vi "Read_Break_List.vi"(8 "error in (no error)":errorcluster, 11 "Ref in":T4={"MS SQL Connection"=refnum, "UDL File"=path "", "Time"="", "DCODE"="", "WIP+1"=0, "MC No?"=0, "POKAYOKE?"=FALSE, "Expected Result"="", "Result [Status]"="", "Clock"=0.0, "RFID"="", "WIP Queue"=refnum, "TS Parameter"={"ProfitCenterCode"="", "LineCode"="", "WorkOrderNumber"="", "Model"="", "Model_with_Prefix"="", "VendorCode"="", "SetParameterDateCode"="", "PokaYoke"=0, "Target"=1, "Live_DateCode"="", "CustomerPartNumber"="", "Hand"="", "sBarcode"=FALSE, "FCA"=0, "Ent_Stamp"=timestamp(0 s since 1904-01-01), "STS_CD"=0.0}, "Data_Queue"=[], "RFID Serial No."=""} {"TS Parameter"."FCA" format="%01d"; "TS Parameter"."Target" min=1 max=100000; "TS Parameter"."PokaYoke" min=0 max=1}) -> (0 "error out":errorcluster, 3 "Break List":T3[](array[typedef]) {"End Time" format="%<%d/%m/%Y\n%I:%M:%S %p>T"; "Start Time" format="%<%d/%m/%Y\n%I:%M:%S %p>T"}, 4 "Operator List":string[](array[string]), 6 "Breakdown List":string[](array[string]))   [LabVIEW 2020]
uses:
  Controls/TD SQL.ctl
  <vilib>/addons/database/Connection.llb/Conn ObjectReference.ctl
  Controls/WIP_State.ctl
  Controls/TS_Parameter.ctl
  Controls/Breakdown_List.ctl
  Controls/Loss_type.ctl
  <vilib>/addons/database/_DB Variant To Data/Database Variant To Data.xnode
  <vilib>/addons/database/NI_Database_API.lvlib
panel:
  out "data 2":string[][](array[string])
  out "f":T1
  out "data":string[](array[string])
  in  "Machine":T2(ring)
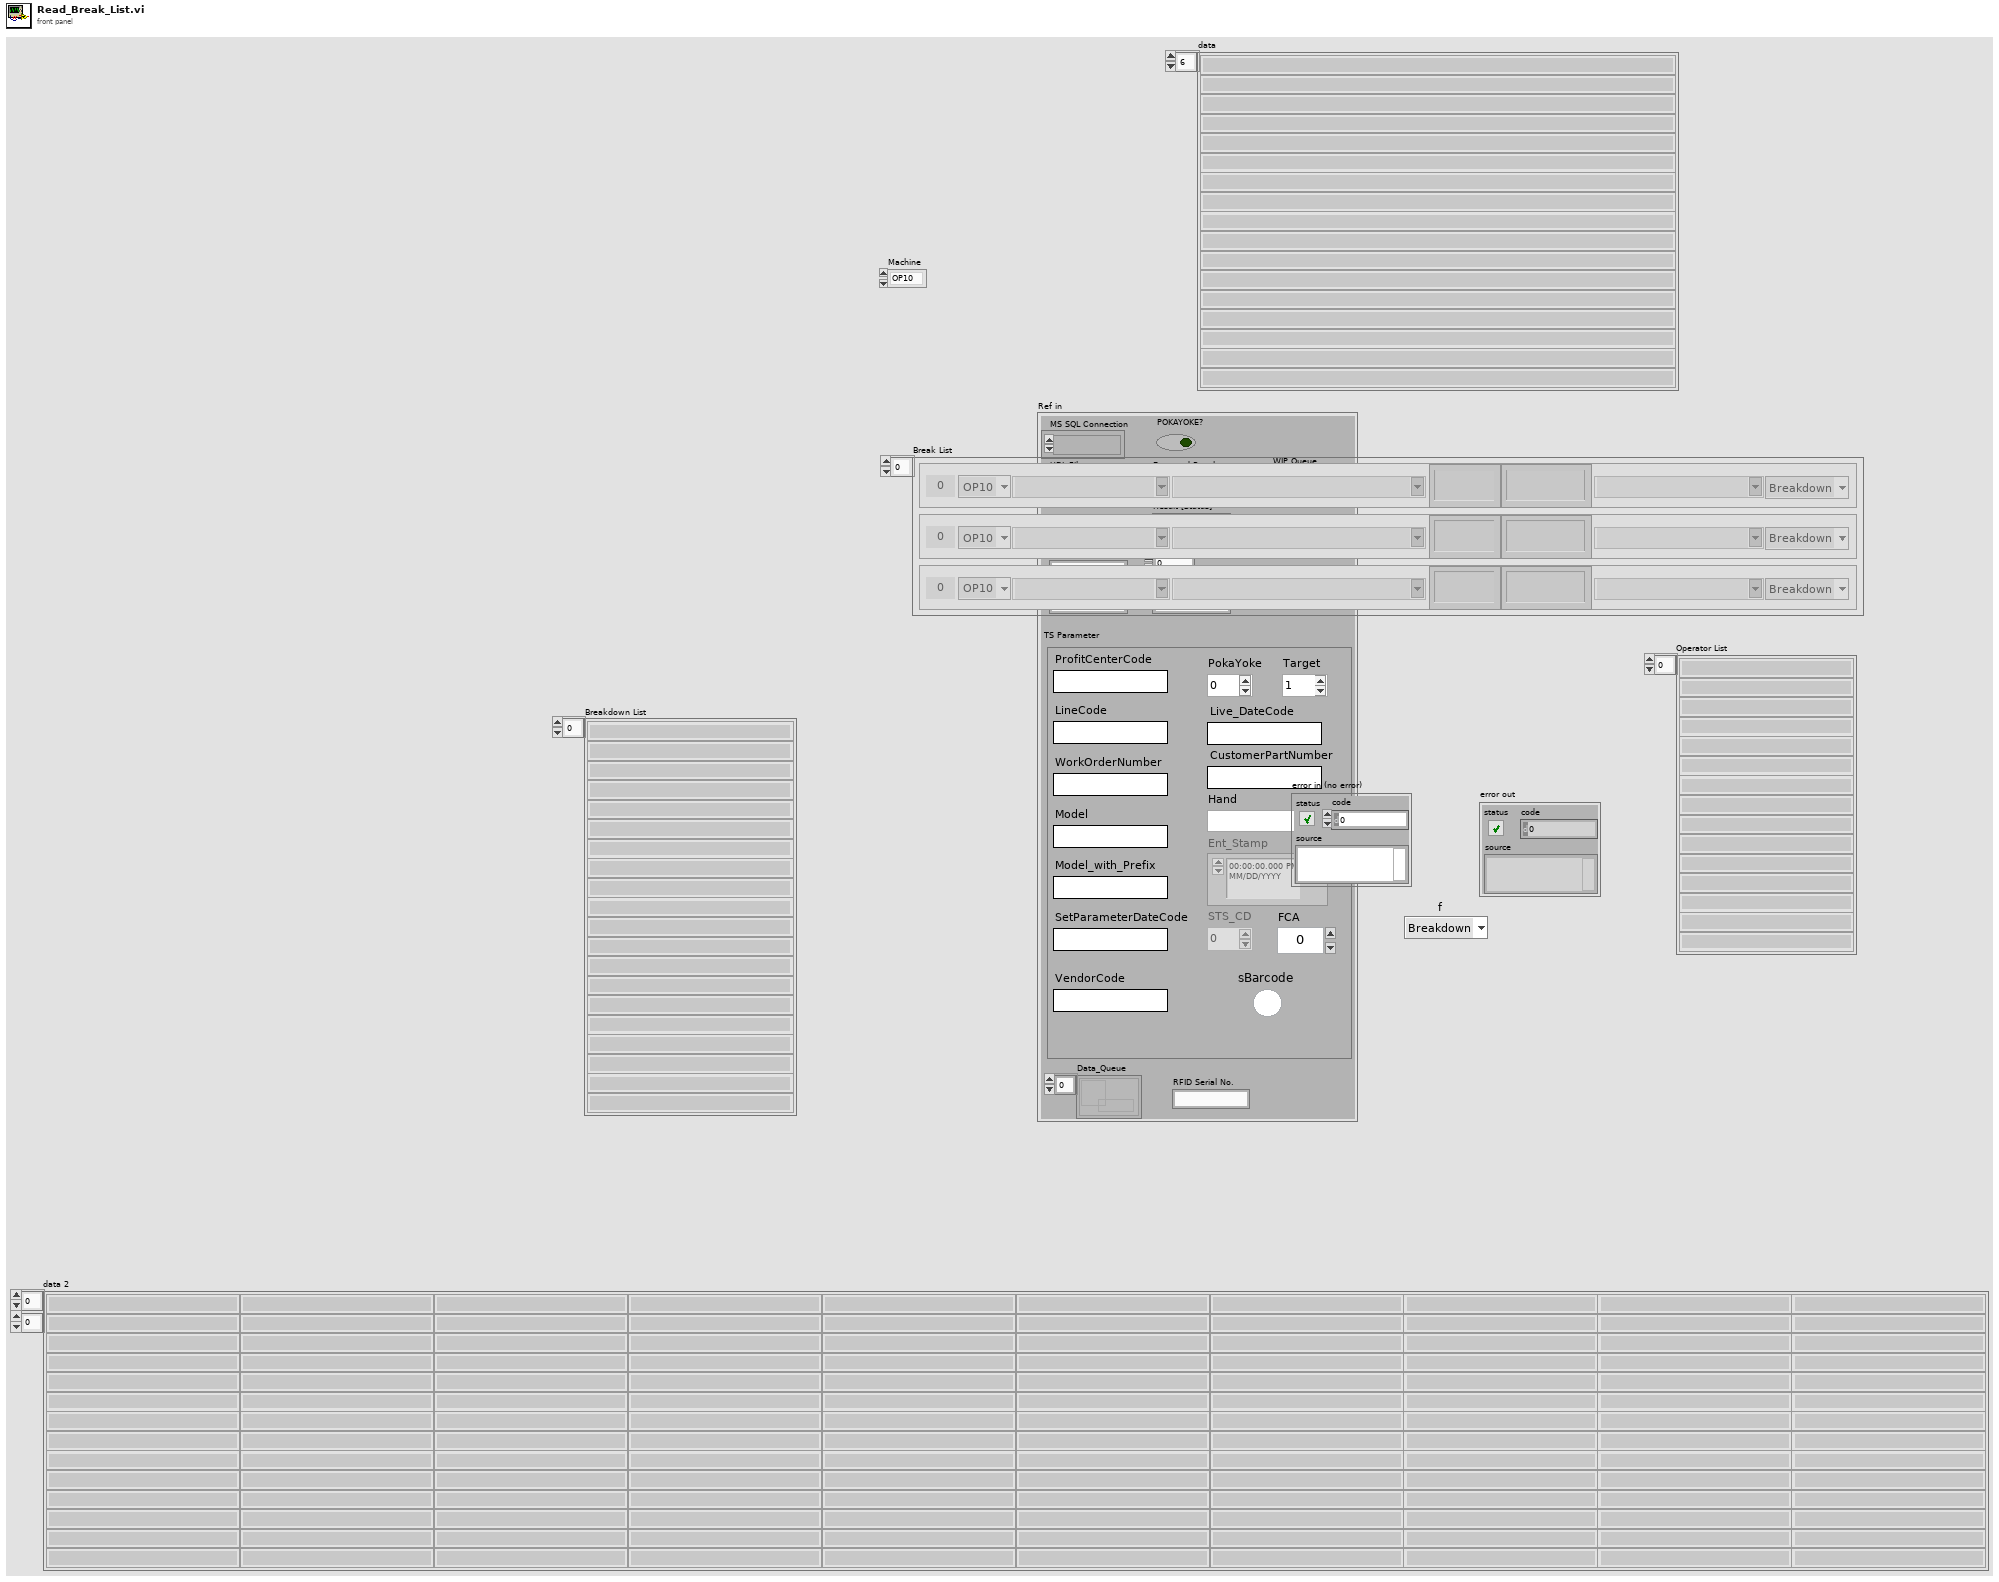
[diagram p1: front panel]
types:
  T1 = typedef "Loss_type.ctl" = enum16{"Breakdown", "Bookout"}
  T2 = enum16{"OP10", "OP20", "OP30", "OP40", "OP50", "OP60", "OP70", "OP80", "LINE"}
  T3 = typedef "Breakdown_List.ctl" = cluster{"S.No":i32, "Reason Code":string, "Start Time":timestamp, "End Time":timestamp, "Operator":string, "Type":T1, "Machine":enum16{"OP10", "OP20", "OP30", "OP40", "OP50", "OP60", "OP70", "OP80", "LINE"}, "Reason":string}
  T4 = typedef "TD SQL.ctl" = cluster{"MS SQL Connection":T5, "UDL File":path, "Time":string, "DCODE":string, "WIP+1":i64, "MC No?":i32, "POKAYOKE?":bool, "Expected Result":string, "Result [Status]":string, "Clock":dbl, "RFID":string, "WIP Queue":refnum<queue>, "TS Parameter":T6, "Data_Queue":refnum<queue>[], "RFID Serial No.":string}
  T5 = typedef "NI_Database_API.lvlib/Conn ObjectReference.ctl" = refnum<k1>
  T6 = typedef "TS_Parameter.ctl" = cluster{"ProfitCenterCode":string, "LineCode":string, "WorkOrderNumber":string, "Model":string, "Model_with_Prefix":string, "VendorCode":string, "SetParameterDateCode":string, "PokaYoke":i32, "Target":i32, "Live_DateCode":string, "CustomerPartNumber":string, "Hand":string, "sBarcode":bool, "FCA":i32, "Ent_Stamp":timestamp, "STS_CD":dbl}
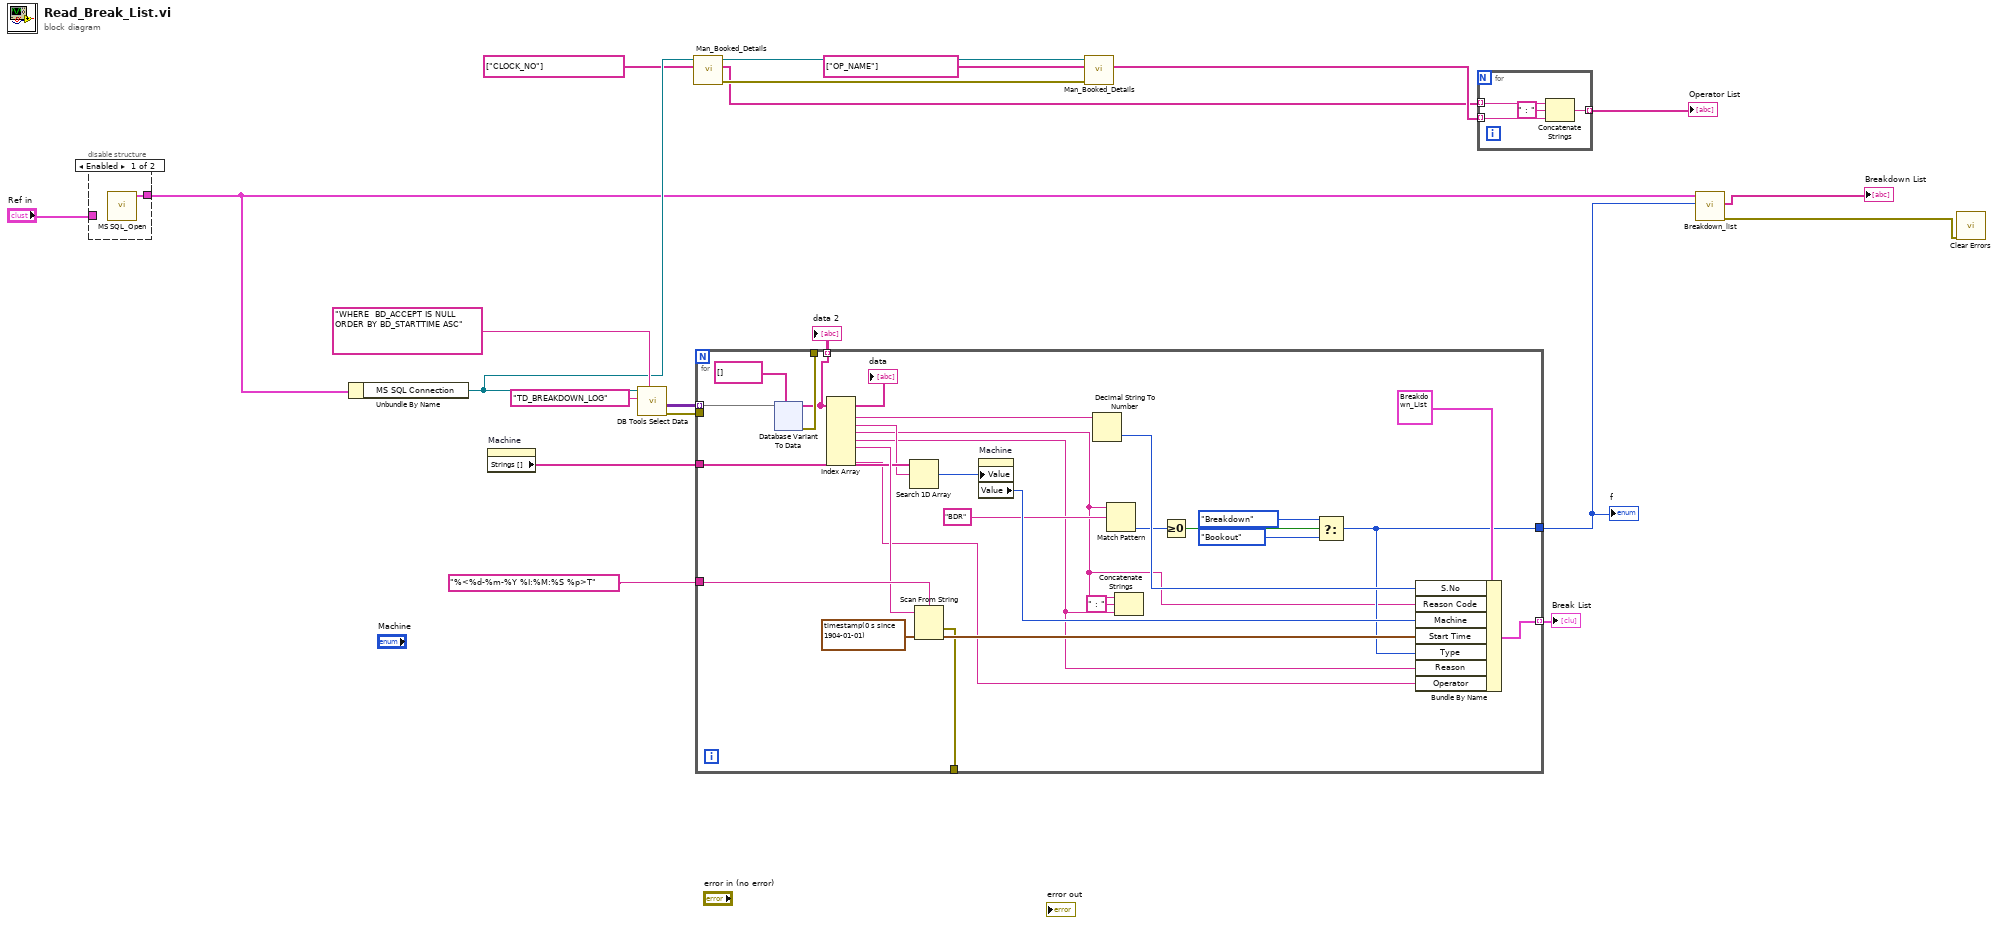
[diagram p0: block diagram]
diagram:
  n1 = disable-structure shown="Enabled" {
    disable-tunnel: [w22 w23] -> w2
    disable-tunnel: "Ref in" -> [_ w23]
    frame Enabled {
      n2 = call "MS SQL_Open.vi"() -> ("Ref Out"=w22:T4)  [unwired: 9 in, 2 out]
    }
    frame Disabled {
    }
  }
  n3 = Unbundle By Name(w2) -> ("MS SQL Connection"=w12:T5)
  n4 = property on="Machine" class="Enum (strict)"() -> ("Strings []"=w7:string[])  [unwired: 2 in, 2 out]
  n5 = call <vilib>:"DB Tools Select Data.vi"("condition"="WHERE  BD_ACCEPT IS NULL ORDER BY BD_STARTTIME ASC", "table"="TD_BREAKDOWN_LOG", "connection reference"=w12) -> ("error out"=w16:errorcluster, "data"=w19:variant[][])  [unwired: 3 in, 1 out]
  n6 = call "Man_Booked_Details.vi"("Column"=string[] ["CLOCK_NO"] ("array"), "Refnum in"=w12) -> ("error out"=w14:errorcluster, "Data"=w8:string[], "Refnum Out"=w15:T5)  [unwired: 7 in]
  n7 = for {
    tunnel: w19 -> [w50] mode=indexing
    tunnel: "%<%d-%m-%Y %I:%M:%S %p>T" ("time format string (%c)") -> [w47]
    tunnel: [w45] -> w17 mode=indexing
    tunnel: [w44] -> _
    tunnel: w16 -> [_]
    tunnel: w7 -> [w41]
    tunnel: [w39] -> _
    tunnel: [w28] -> w5
    tunnel: [w24] -> w3 mode=indexing
    n8 = xnode "Database Variant To Data"("database variant"=w50, "type"=string[] []) -> ("data"=w24:string[], "error out"=w39:errorcluster)  [unwired: 1 in]
    "data" <- w24
    n9 = Index Array(array=w24) -> (element #1=w43:string, element #2=w40:string, element #3=w27:string, element #4=w26:string, element #5=w42:string, element #7=w25:string)  [unwired: 7 in, 1 out]
    n10 = Search 1D Array(1D array=w41, element=w40) -> (index of element=w38:i32)  [unwired: 1 in]
    n11 = Scan From String(format string=w47, input string=w42, default 1=timestamp(0 s since 1904-01-01) ("default value 1")) -> (error out=w44:errorcluster, output 1=w46:timestamp)  [unwired: 2 in, 2 out]
    n12 = property on="Machine" class="Enum (strict)"("Value"=w38) -> ("Value"=w37:T2)  [unwired: 2 in, 2 out]
    n13 = Decimal String To Number(string=w43) -> (number=w36:i32)  [unwired: 2 in, 1 out]
    n14 = Match Pattern(string=w27, regular expression="BDR") -> (offset past match=w32:i32)  [unwired: 1 in, 3 out]
    n15 = Concatenate Strings(w27, " : " ("string"), w26) -> ()  [unwired: 1 out]
    n16 = Greater Or Equal To 0?(x=w32) -> (x >= 0?=w31:bool)
    n17 = Select(t=Loss_type."Breakdown" ("Type"), s=w31, f=Loss_type."Bookout") -> (s? t:f=w28:T1)
    n18 = Bundle By Name(cluster=T3 {"S.No"=0, "Reason Code"="", "Start Time"=timestamp(0 s since 1904-01-01), "End Time"=timestamp(0 s since 1904-01-01), "Operator"="", "Type"=enum."Bookout", "Machine"=enum."OP10", "Reason"=""} ("Bootout"), "S.No"=w36, "Reason Code"=w27, "Machine"=w37, "Start Time"=w46, "Type"=w28, "Reason"=w26, "Operator"=w25) -> (w45:T3)
  }
  "Break List" <- w17
  "f" <- w5
  "data 2" <- w3
  n19 = call "Man_Booked_Details.vi"("error in (no error)"=w14, "Column"=string[] ["OP_NAME"] ("array"), "Refnum in"=w15) -> ("Data"=w10:string[])  [unwired: 6 in, 2 out]
  n20 = for {
    tunnel: w8 -> [w92] mode=indexing
    tunnel: w10 -> [w91] mode=indexing
    tunnel: [w89] -> w9 mode=indexing
    n21 = Concatenate Strings(w92, " : " ("string"), w91) -> (w89:string)
  }
  "Operator List" <- w9
  n22 = call "Breakdown_list.vi"("Reason Type"=w5, "Ref In"=w2) -> ("error out"=w6:errorcluster, "Reason List"=→"Breakdown List":string[])  [unwired: 6 in, 2 out]
  n23 = call <vilib>:"Clear Errors.vi"("error in (no error)"=w6) -> ()  [unwired: 5 in, 2 out]
